vi "to string.vi"(8 "error in":errorcluster, 11 "Tagbus PID Module configuration in":refnum<class "PID Module configuration.lvclass">) -> (0 "error out":errorcluster, 1 "data":string, 2 "version":string, 3 "Tagbus PID Module configuration out":refnum<class "PID Module configuration.lvclass">)   [LabVIEW 2013, in "PID Module configuration.lvclass"]
doc: "Provides an interface for saving a module configuration to a file or other serialized data source. It is recommended that all children of this class store data in two sets--data required for its own initialization, and any data required for parent initialization--and that each implementation uses the <b>Call Parent Method</b> primitive to serialize parent information."
uses:
  PID Module configuration.lvclass
  <vilib>/NI/Tag Bus Module Framework/module configuration/TBM module configuration.lvclass
  PID Module configuration.lvclass/PID Module configuration.ctl
  PID Loop.lvclass
  current version.vi
  <vilib>/NI/Configuration Framework/serializable configuration/NISE_CEF_serializable configuration.lvclass
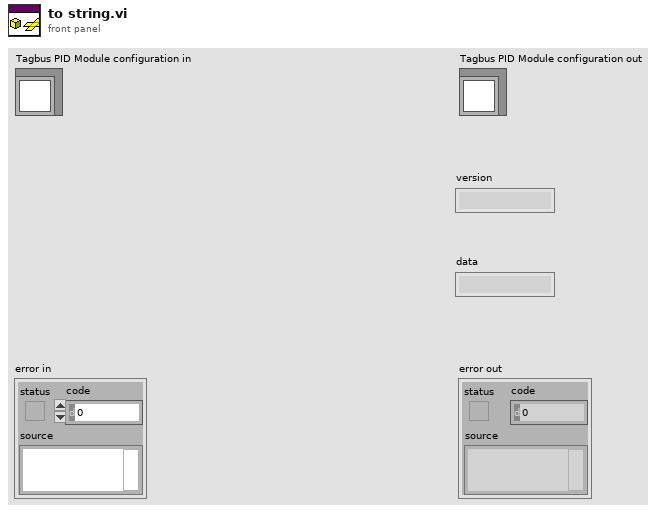
[diagram p1: front panel]
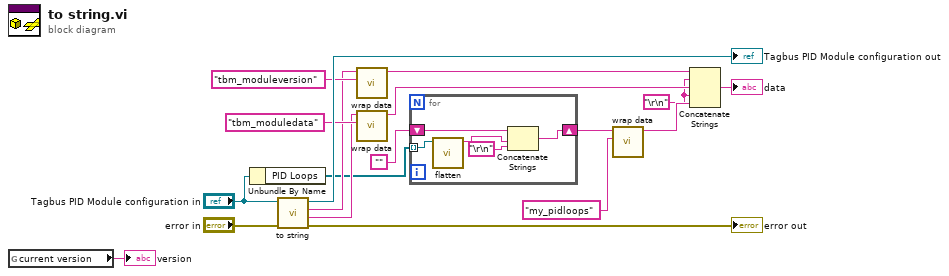
[diagram p0: block diagram]
diagram:
  w3 = "\r\n"
  n1 = global read "current version.vi" "current version"() -> (→"version":string)
  n2 = Unbundle By Name("Tagbus PID Module configuration in") -> ("PID Loops"=w1:refnum<class "PID Loop.lvclass">[])
  n3 = call-parent "to string.vi"("error in"="error in", "module configuration in"="Tagbus PID Module configuration in") -> ("error out"=→"error out":errorcluster, "data"=w9:string, "version"=w10:string, "module configuration out"=→"Tagbus PID Module configuration out":refnum<class "PID Module configuration.lvclass">)  [unwired: 6 in]
  n4 = call <vilib>:"wrap data.vi"("identifier"="tbm_moduleversion" ("additional identifier"), "data to wrap"=w10) -> ("wrapped data"=w12:string)  [unwired: 9 in]
  n5 = call <vilib>:"wrap data.vi"("identifier"="tbm_moduledata" ("additional identifier"), "data to wrap"=w9) -> ("wrapped data"=w11:string)  [unwired: 9 in]
  n6 = for {
    shift-right: [w22] -> w4
    shift-left: "" -> [w21]
    tunnel: w1 -> [w20] mode=indexing
    n7 = call-dynamic "flatten.vi"("PID Loop in"=w20) -> ("flattened PID Loop"=w19:string)  [unwired: 9 in, 1 out]
    n8 = Concatenate Strings(w21, w19, "\r\n") -> (w22:string)
  }
  n9 = call <vilib>:"wrap data.vi"("identifier"="my_pidloops" ("additional identifier"), "data to wrap"=w4) -> ("wrapped data"=w7:string)  [unwired: 9 in]
  n10 = Concatenate Strings(w12, w3, w11, w3, w7) -> (→"data":string)
